vi "Lab10.vi"() -> ()   [LabVIEW 2022 SP3]
uses:
  <vilib>/DAQmx/write.llb/DAQmx Write (Digital 1D Bool 1Chan 1Samp).vi
  <vilib>/DAQmx/create/channels.llb/DAQmx Create Channel (DO-Digital Output).vi
  <vilib>/DAQmx/miscellaneous.llb/DAQmx Fill In Error Info.vi
panel:
  in  "stop":bool
  in  "Array":bool[](array[boolean])
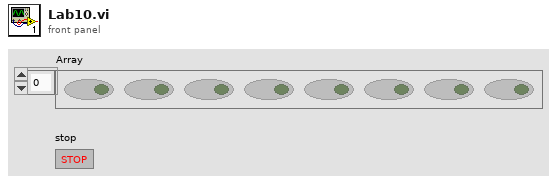
[diagram p1: front panel]
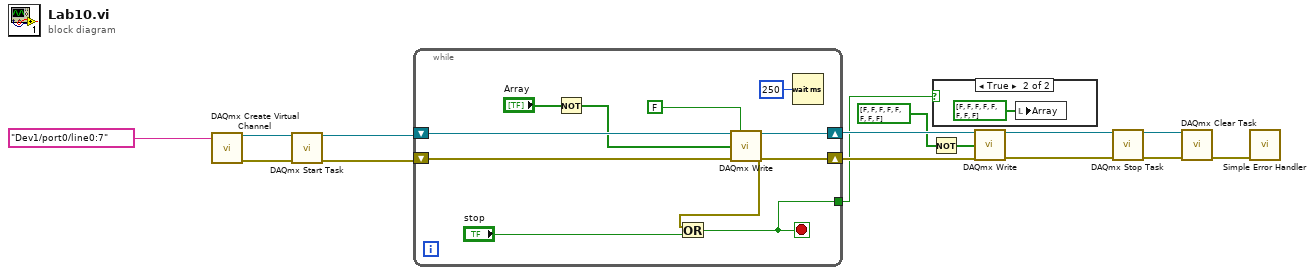
[diagram p0: block diagram]
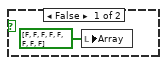
[diagram p2: hidden frame]
diagram:
  n1 = call-poly <vilib>:"DAQmx Create Virtual Channel.vi"("lines"=tag "Dev1/port0/line0:7") -> ("task out"=w15:refnum<k21>, "error out"=w14:errorcluster)  [unwired: 13 in]
  n2 = call <vilib>:"DAQmx Start Task.vi"("task/channels in"=w15, "error in"=w14) -> ("task out"=w13:refnum<k21>, "error out"=w12:errorcluster)  [unwired: 12 in]
  n3 = while {
    shift-right: [w20] -> w7
    shift-left: w13 -> [w24]
    shift-right: [w17] -> w6
    shift-left: w12 -> [w25]
    tunnel: [w16] -> w1
    stop <- w16 stop-if-true
    n4 = Not(x="Array") -> (.not. x?=w18:bool[])
    n5 = call-poly <vilib>:"DAQmx Write.vi"("task/channels in"=w24, "auto start"=FALSE, "data"=w18, "error in"=w25) -> ("task out"=w20:refnum<k21>, "error out"=w17:errorcluster)  [unwired: 9 in, 1 out]
    n6 = Or(x=w17, y="stop") -> (x .or. y?=w16:bool)
    n7 = Wait (ms)(milliseconds to wait=u32 250) -> ()  [unwired: 1 out]
  }
  n8 = Not(x=bool[] [FALSE, FALSE, FALSE, FALSE, FALSE, FALSE, FALSE, FALSE] ("Array")) -> (.not. x?=w3:bool[])
  n9 = case shown="True" w1 {
    frame False {
      n10 = local write "Array"(bool[] [FALSE, FALSE, FALSE, FALSE, FALSE, FALSE, FALSE, FALSE] ("Array")) -> ()
    }
    frame True {
      n11 = local write "Array"(bool[] [FALSE, FALSE, FALSE, FALSE, FALSE, FALSE, FALSE, FALSE] ("Array")) -> ()
    }
  }
  n12 = call-poly <vilib>:"DAQmx Write.vi"("task/channels in"=w7, "data"=w3, "error in"=w6) -> ("task out"=w5:refnum<k21>, "error out"=w4:errorcluster)  [unwired: 10 in, 1 out]
  n13 = call <vilib>:"DAQmx Stop Task.vi"("task/channels in"=w5, "error in"=w4) -> ("task out"=w10:refnum<k21>, "error out"=w11:errorcluster)  [unwired: 12 in]
  n14 = call <vilib>:"DAQmx Clear Task.vi"("task in"=w10, "error in"=w11) -> ("error out"=w9:errorcluster)  [unwired: 13 in]
  n15 = call <vilib>:"Simple Error Handler.vi"("error in (no error)"=w9) -> ()  [unwired: 4 in, 5 out]
